vi "Dialog.vi"(7 "Open? [T]":bool=TRUE, 8 "error in (no error)":errorcluster) -> ()   [LabVIEW 2020, in "Multiple Errors.lvclass"]
uses:
  Multiple Errors.lvclass
panel:
  out "Warning":string="WARNING: Only the first 1000 errors are listed!"
  in  "Error":string
  in  "Items":i32(c297)
  out "Item":string
  out "Acknowledged":bool
  in  "OK":bool
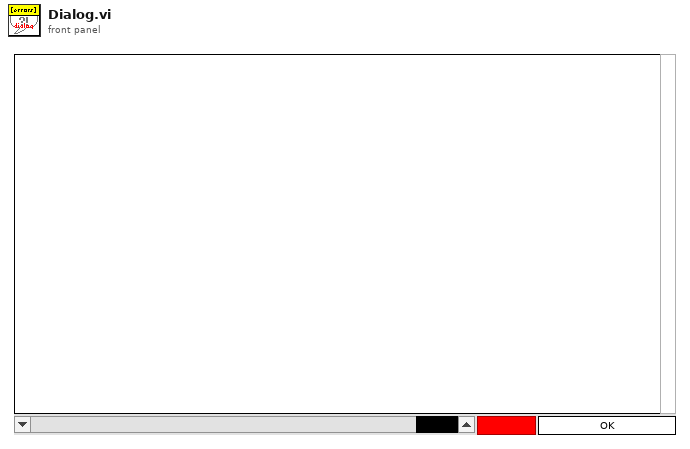
[diagram p1: front panel]
types:
  T1 = enum32{"Invalid", "Standard", "Closed", "Hidden", "Minimized", "Maximized"}
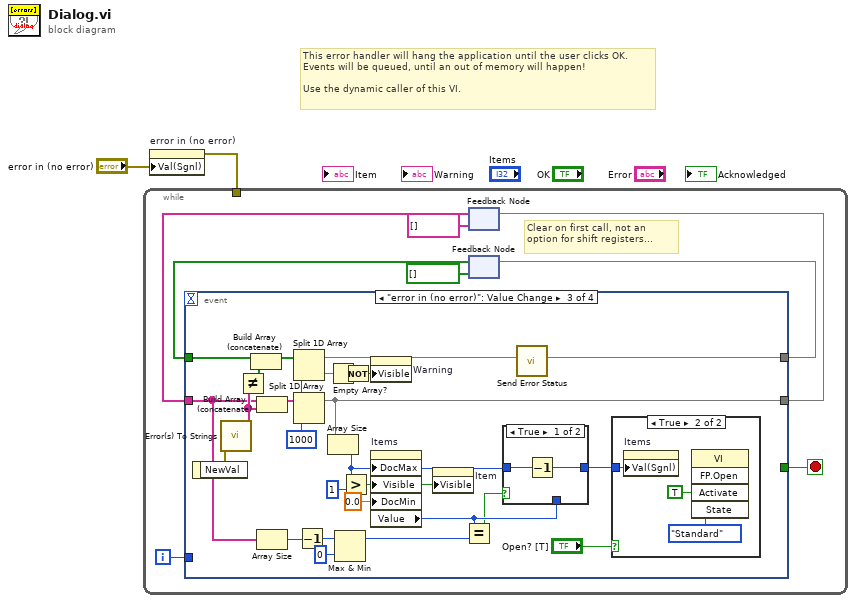
[diagram p0: block diagram]
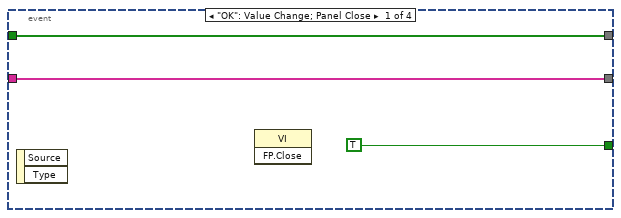
[diagram p2: hidden frame]
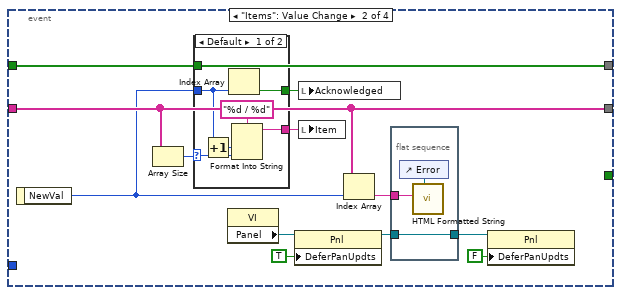
[diagram p3: hidden frame]
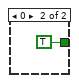
[diagram p4: hidden frame]
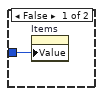
[diagram p6: hidden frame]
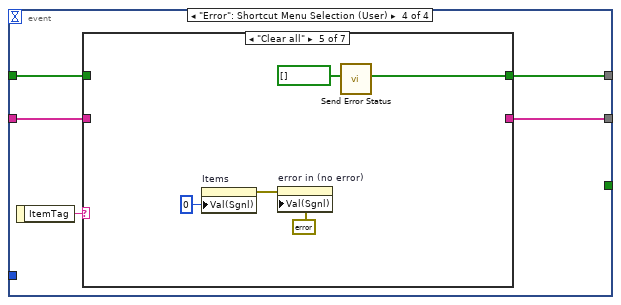
[diagram p7: hidden frame]
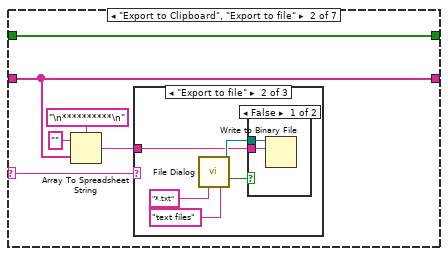
[diagram p9: hidden frame]
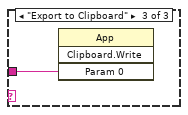
[diagram p12: hidden frame]
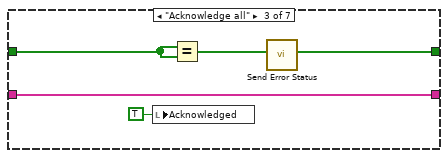
[diagram p13: hidden frame]
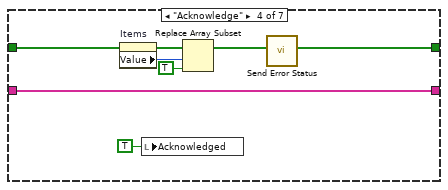
[diagram p14: hidden frame]
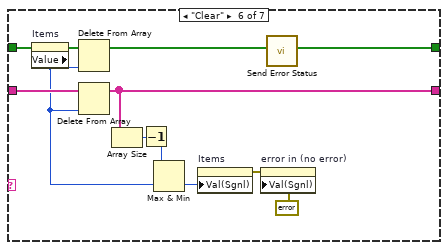
[diagram p15: hidden frame]
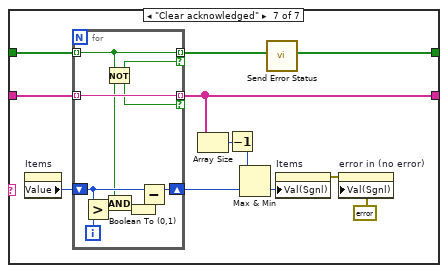
[diagram p16: hidden frame]
diagram:
  # "This error handler will hang the application until the user clicks OK.\nEvents will be queued, until an out of memory will happen!\n\nUse the dynamic caller of this VI."
  n1 = property on="error in (no error)" class="Clust (strict)"("Val(Sgnl)"="error in (no error)") -> (error out=w1:errorcluster)  [unwired: 2 in, 1 out]
  n2 = while {
    tunnel: w1 -> [_]
    i -> [w9]
    stop <- w10 stop-if-true
    # "Clear on first call, not an option for shift registers..."
    n3 = feedback #1(string[] []) -> (w5:string[])
    n4 = feedback #2(bool[] []) -> (w7:bool[])
    n5 = event shown="[2] \"error in (no error)\": Value Change" {
      selector: _ -> [_ _ _ _]
      dyn-events: _ -> [_ _ _ _]
      timeout: _ -> [_ _ _ _]
      tunnel: [TRUE _ _ _] -> w10
      tunnel: w5 -> [w12 w19 w43 w73]
      tunnel: [w12 w19 w55 w71] -> w6
      tunnel: w9 -> [_ _ _ _]
      tunnel: w7 -> [w11 w17 w50 w69]
      tunnel: [w11 w17 w51 w70] -> w8
      event "OK": Value Change; Panel Close {
        n6 = event-data() -> ()  [unwired: 1 in, 2 out]
        n7 = invoke class="VI" method="FP.Close"() -> ()  [unwired: 3 in, 3 out]
      }
      event "Items": Value Change {
        n8 = event-data() -> ("NewVal"=w14:i32)  [unwired: 1 in]
        n9 = Array Size(array=w19) -> (size(s)=w15:i32)
        n10 = case shown="Default" w15 {
          selector: w15 -> [w32 _]
          tunnel: [w30 _] -> w18
          tunnel: w17 -> [w29 _]
          tunnel: w14 -> [w26 _]
          tunnel: [w28 TRUE ("Boolean")] -> w16
          frame Default {
            n11 = Increment(x=w26) -> (x+1=w27:i32)
            n12 = Index Array(array=w29, index=w26) -> (element=w28:bool)
            n13 = Format Into String(format string="%d / %d", w27, w32) -> (resulting string=w30:string)  [unwired: 2 in, 1 out]
          }
          frame 0 {
          }
        }
        n14 = property class="VI"() -> ("Panel"=w24:refnum<vi>)  [unwired: 2 in, 2 out]
        n15 = property class="Pnl"(reference=w24, "DeferPanUpdts"=TRUE ("Defer Panel Updates")) -> (reference out=w23:refnum<vi>)  [unwired: 1 in, 1 out]
        n16 = local write "Acknowledged"(w16) -> ()
        n17 = local write "Item"(w18) -> ()
        n18 = Index Array(array=w19, index=w14) -> (element=w25:string)
        n19 = flat-sequence {
          tunnel: w25 -> [w36]
          tunnel: w23 -> [w34]
          tunnel: [w34] -> w22
          frame #0 {
            n20 = control-ref of="Error"() -> (w35:refnum<vi>)
            n21 = call "HTML Formatted String.vi"("Str Refnum"=w35, "Message"=w36) -> ()  [unwired: 10 in]
          }
        }
        n22 = property class="Pnl"(reference=w22, "DeferPanUpdts"=FALSE ("Defer Panel Updates")) -> ()  [unwired: 1 in, 2 out]
      }
      event "error in (no error)": Value Change {
        w53 = 1000 ("length")
        n23 = event-data() -> ("NewVal"=w47:errorcluster)  [unwired: 1 in]
        n24 = call "Error(s) To Strings.vi"("error in (no error)"=w47) -> ("Error Strings"=w52:string[])  [unwired: 10 in]
        n25 = Not Equal?(x=w52, y=w52) -> (x != y?=w49:bool[])
        n26 = Build Array (concatenate)(w50, w49) -> (w54:bool[])
        n27 = Build Array (concatenate)(w43, w52) -> (w59:string[])
        n28 = Array Size(array=w43) -> (size(s)=w42:i32)
        n29 = Split 1D Array(array=w54, index=w53) -> (first subarray=w51:bool[], second subarray=w48:bool[])
        n30 = Split 1D Array(array=w59, index=w53) -> (first subarray=w55:string[])  [unwired: 1 out]
        n31 = Decrement(x=w42) -> (x-1=w41:i32)
        n32 = Empty Array?(array=w48) -> (empty?=w58:bool)
        n33 = Array Size(array=w55) -> (size(s)=w45:i32)
        n34 = Max & Min(x=w41, y=0) -> (max(x,y)=w38:i32)  [unwired: 1 out]
        n35 = Greater?(x=w45, y=1 ("x")) -> (0:w56:bool)
        n36 = Not(x=w58) -> (.not. x?=w57:bool)
        n37 = property on="Warning" class="Str"("Visible"=w57) -> ()  [unwired: 2 in, 2 out]
        n38 = property on="Items" class="Scroll (strict)"("DocMax"=w45, "Visible"=w56, "DocMin"=0.0 ("Doc Min")) -> ("Value"=w40:i32)  [unwired: 2 in, 2 out]
        n39 = property on="Item" class="Str"("Visible"=w56) -> ()  [unwired: 2 in, 2 out]
        n40 = Equal?(x=w40, y=w38) -> (x = y?=w39:bool)
        n41 = case shown="True" w39 {
          tunnel: w40 -> [_ w64]
          tunnel: [w62 w64] -> w44
          tunnel: w45 -> [w63 _]
          frame True {
            n42 = Decrement(x=w63) -> (x-1=w62:i32)
          }
          frame False {
          }
        }
        n43 = call "Send Error Status.vi"("Errors"=w51) -> ()  [unwired: 11 in]
        n44 = case shown="True" "Open? [T]" {
          tunnel: w44 -> [w65 w66]
          frame False {
            n45 = property on="Items" class="Scroll (strict)"("Value"=w65) -> ()  [unwired: 2 in, 2 out]
          }
          frame True {
            n46 = property on="Items" class="Scroll (strict)"("Val(Sgnl)"=w66) -> ()  [unwired: 2 in, 2 out]
            n47 = invoke class="VI" method="FP.Open"("Activate"=TRUE ("Activate?"), "State"=T1."Standard") -> ()  [unwired: 3 in, 5 out]
          }
        }
      }
      event "Error": Shortcut Menu Selection (User) {
        n48 = event-data() -> ("ItemTag"=w72:string)  [unwired: 1 in]
        n49 = case shown="\"Clear all\"" w72 {
          selector: w72 -> [_ w79 _ _ _ _ _]
          tunnel: w73 -> [w74 w77 w93 w99 _ w111 w122]
          tunnel: [w74 w77 w93 w99 _ w109 w120] -> w71
          tunnel: [w75 w76 w90 w95 w103 w112 w123] -> w70
          tunnel: w69 -> [w75 w76 w92 w98 _ w113 w124]
          frame Default {
          }
          frame "Export to Clipboard", "Export to file" {
            n50 = Array To Spreadsheet String(delimiter (Tab)="\n**********\n", array=w77, 3:"" ("format string")) -> (spreadsheet string=w78:string)
            n51 = case shown="\"Export to file\"" w79 {
              tunnel: w78 -> [_ w83 w89]
              frame Default {
              }
              frame "Export to file" {
                n52 = call "File Dialog"("pattern (all files)"="*.txt", "pattern label"="text files") -> ("selected path"=w84:path, "cancelled"=w82:bool)  [unwired: 10 in, 2 out]
                n53 = case shown="False" w82 {
                  tunnel: w84 -> [w88 _]
                  tunnel: w83 -> [w87 _]
                  frame False {
                    n54 = Write to Binary File(file (use dialog)=w88, data=w87) -> ()  [unwired: 4 in, 3 out]
                  }
                  frame True {
                  }
                }
              }
              frame "Export to Clipboard" {
                n55 = invoke class="App" method="Clipboard.Write"("Param 0"=w89) -> ()  [unwired: 3 in, 4 out]
              }
            }
          }
          frame "Acknowledge all" {
            n56 = local write "Acknowledged"(TRUE ("Acknowledged")) -> ()
            n57 = Equal?(x=w92, y=w92) -> (x = y?=w90:bool[])
            n58 = call "Send Error Status.vi"("Errors"=w90) -> ()  [unwired: 11 in]
          }
          frame "Acknowledge" {
            n59 = property on="Items" class="Scroll (strict)"() -> ("Value"=w97:i32)  [unwired: 2 in, 2 out]
            n60 = local write "Acknowledged"(TRUE ("Acknowledged")) -> ()
            n61 = Replace Array Subset(array=w98, new element=TRUE ("new element/subarray"), index=w97) -> (w95:bool[])
            n62 = call "Send Error Status.vi"("Errors"=w95) -> ()  [unwired: 11 in]
          }
          frame "Clear all" {
            w103 = bool[] [] ("Errors")
            n63 = property on="Items" class="Scroll (strict)"("Val(Sgnl)"=0 ("Value (Signaling)")) -> (error out=w101:errorcluster)  [unwired: 2 in, 1 out]
            n64 = property on="error in (no error)" class="Clust (strict)"(error in=w101, "Val(Sgnl)"=errorcluster {"status"=FALSE, "code"=0, "source"=""} ("Value (Signaling)")) -> ()  [unwired: 1 in, 2 out]
            n65 = call "Send Error Status.vi"("Errors"=w103) -> ()  [unwired: 11 in]
          }
          frame "Clear" {
            n66 = property on="Items" class="Scroll (strict)"() -> ("Value"=w104:i32)  [unwired: 2 in, 2 out]
            n67 = Delete From Array(array=w113, index=w104) -> (array with subset deleted=w112:bool[])  [unwired: 1 in, 1 out]
            n68 = Delete From Array(array=w111, index=w104) -> (array with subset deleted=w109:string[])  [unwired: 1 in, 1 out]
            n69 = Array Size(array=w109) -> (size(s)=w108:i32)
            n70 = Decrement(x=w108) -> (x-1=w107:i32)
            n71 = Max & Min(x=w107, y=w104) -> (min(x,y)=w110:i32)  [unwired: 1 out]
            n72 = property on="Items" class="Scroll (strict)"("Val(Sgnl)"=w110) -> (error out=w105:errorcluster)  [unwired: 2 in, 1 out]
            n73 = property on="error in (no error)" class="Clust (strict)"(error in=w105, "Val(Sgnl)"=errorcluster {"status"=FALSE, "code"=0, "source"=""} ("Value (Signaling)")) -> ()  [unwired: 1 in, 2 out]
            n74 = call "Send Error Status.vi"("Errors"=w112) -> ()  [unwired: 11 in]
          }
          frame "Clear acknowledged" {
            n75 = property on="Items" class="Scroll (strict)"() -> ("Value"=w115:i32)  [unwired: 2 in, 2 out]
            n76 = for {
              tunnel: w124 -> [w125] mode=indexing
              tunnel: [w125] -> w123 mode=indexing if=w132
              tunnel: w122 -> [w133] mode=indexing
              tunnel: [w133] -> w120 mode=indexing if=w132
              shift-right: [w128] -> w114
              shift-left: w115 -> [w130]
              i -> [w131]
              n77 = Greater?(x=w130, y=w131) -> (0:w127:bool)
              n78 = Not(x=w125) -> (.not. x?=w132:bool)
              n79 = And(x=w125, y=w127) -> (x .and. y?=w126:bool)
              n80 = Boolean To (0,1)(Boolean=w126) -> (0, 1=w129:i16)
              n81 = Subtract(x=w130, y=w129) -> (x-y=w128:i32)
            }
            n82 = Array Size(array=w120) -> (size(s)=w119:i32)
            n83 = Decrement(x=w119) -> (x-1=w118:i32)
            n84 = Max & Min(x=w118, y=w114) -> (min(x,y)=w121:i32)  [unwired: 1 out]
            n85 = call "Send Error Status.vi"("Errors"=w123) -> ()  [unwired: 11 in]
            n86 = property on="Items" class="Scroll (strict)"("Val(Sgnl)"=w121) -> (error out=w116:errorcluster)  [unwired: 2 in, 1 out]
            n87 = property on="error in (no error)" class="Clust (strict)"(error in=w116, "Val(Sgnl)"=errorcluster {"status"=FALSE, "code"=0, "source"=""} ("Value (Signaling)")) -> ()  [unwired: 1 in, 2 out]
          }
        }
      }
    }
    n88 = feedback-in #1(w6) -> ()
    n89 = feedback-in #2(w8) -> ()
  }
